vi "Fire_Motor.vi"   [LabVIEW 2011]
uses:
  StateMachineType.ctl
  Robot Global Data.vi
types:
  T1 = typedef "StateMachineType.ctl" = enum16{"Init", "Idle", "Start", "Do", "Stop"}
  T2 = typedef "WPI_MotorControlDeviceRef.ctl" = cluster{"DeviceStatus":errorcluster, "Type":enum16{"PWM", "CAN"}, "PWM":cluster{"Digital Module":T3, "PWM Channel":T4, "DeadBand":T5}, "CAN":cluster{"Device Number":u8, "Control Mode":T6, "Semaphore":T7, "Max Vout":dbl}, "Invert":bool, "TransformRef":T8, "InvTransformRef":T8}
  T3 = typedef "FPGA_TypedefDigitalModule.ctl" = enum16{"Digital Module 1", "Digital Module 2"}
  T4 = typedef "FPGA_DIOPWMChannel.ctl" = enum8{"PWM 1", "PWM 2", "PWM 3", "PWM 4", "PWM 5", "PWM 6", "PWM 7", "PWM 8", "PWM 9", "PWM 10", "Invalid"}
  T5 = typedef "WPI_PWMDeadband.ctl" = cluster{"Name":string, "maxPositivePwm":i32, "minPositivePwm":i32, "centerPwm":i32, "maxNegativePwm":i32, "minNegativePwm":i32, "angularRange":u16}
  T6 = typedef "WPI_CANJaguar_ControlMode.ctl" = enum8{"Percent VBus", "Current", "Speed", "Position", "Voltage"}
  T7 = typedef "Semaphore RefNum" = refnum<k1>
  T8 = typedef "WPI_PWMTransform_ConPane.ctl" = refnum<vi>
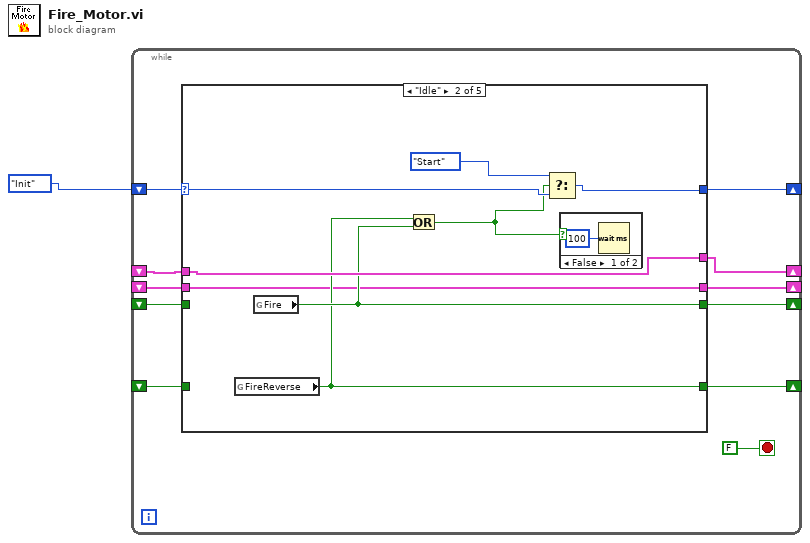
[diagram p0: block diagram]
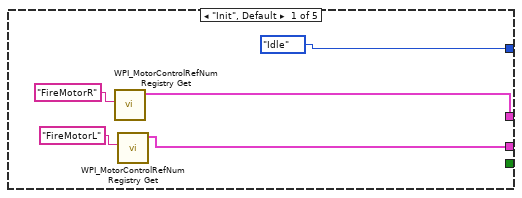
[diagram p2: hidden frame]
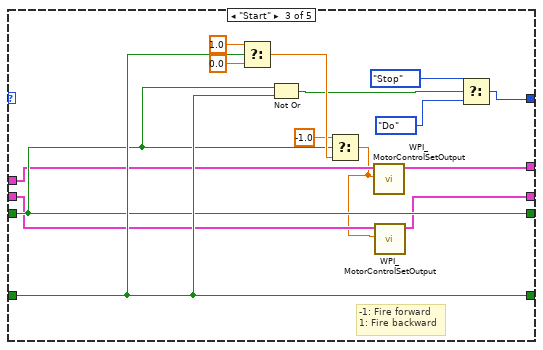
[diagram p4: hidden frame]
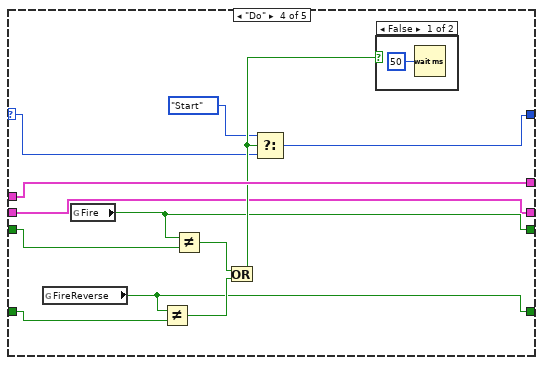
[diagram p5: hidden frame]
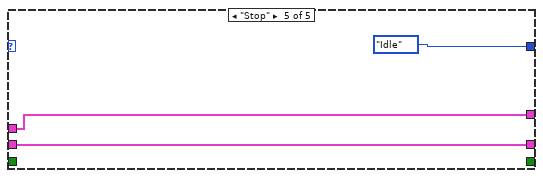
[diagram p7: hidden frame]
diagram:
  n1 = while {
    shift-right: [w8] -> _
    shift-left: _ -> [w11]
    shift-right: [w9] -> _
    shift-left: StateMachineType."Init" -> [w10]
    shift-right: [w6] -> _
    shift-left: _ -> [w4]
    shift-right: [w7] -> _
    shift-left: _ -> [w5]
    shift-right: [w3] -> _
    shift-left: _ -> [w2]
    stop <- FALSE stop-if-true
    n2 = case shown="\"Idle\"" w10 {
      selector: w10 -> [_ w25 _ w43 _]
      tunnel: w11 -> [_ w22 w30 w53 w56]
      tunnel: [StateMachineType."Idle" ("Enum") w23 w37 w47 StateMachineType."Idle" ("Enum")] -> w9
      tunnel: [w15 w22 w41 w53 w56] -> w8
      tunnel: [_ w20 w34 w46 _] -> w7
      tunnel: [_ w19 w35 w45 _] -> w6
      tunnel: w5 -> [_ _ w34 w52 _]
      tunnel: w4 -> [_ _ w35 w51 _]
      tunnel: [w13 w18 w28 w42 w55] -> w3
      tunnel: w2 -> [_ w18 w29 w42 w55]
      frame "Init", Default {
        n3 = call <vilib>:"WPI_MotorControlRefNum Registry Get.vi"("refnum name"="FireMotorR") -> ("MotorControlDevRef"=w15:T2)  [unwired: 9 in, 1 out]
        n4 = call <vilib>:"WPI_MotorControlRefNum Registry Get.vi"("refnum name"="FireMotorL") -> ("MotorControlDevRef"=w13:T2)  [unwired: 9 in, 1 out]
      }
      frame "Idle" {
        n5 = global read "Robot Global Data.vi" "FireReverse"() -> (w19:bool)
        n6 = global read "Robot Global Data.vi" "Fire"() -> (w20:bool)
        n7 = Or(x=w19, y=w20) -> (x .or. y?=w21:bool)
        n8 = Select(t=StateMachineType."Start" ("Enum"), s=w21, f=w25) -> (s? t:f=w23:T1)
        n9 = case shown="False" w21 {
          frame False {
            n10 = Wait (ms)(milliseconds to wait=u32 100) -> ()  [unwired: 1 out]
          }
          frame True {
          }
        }
      }
      frame "Start" {
        # "-1: Fire forward\n1: Fire backward"
        n11 = Select(t=1.0, s=w35, f=0.0) -> (s? t:f=w40:dbl)
        n12 = Not Or(1:w35, 2:w34) -> (0:w36:bool)
        n13 = Select(t=-1.0, s=w34, f=w40) -> (s? t:f=w27:dbl)
        n14 = call <vilib>:"WPI_MotorControlSetOutput.vi"("Output"=w27, "MotorControlDevRef"=w30) -> ("MotorControlDevRef"=w41:T2)  [unwired: 8 in, 1 out]
        n15 = call <vilib>:"WPI_MotorControlSetOutput.vi"("Output"=w27, "MotorControlDevRef"=w29) -> ("MotorControlDevRef"=w28:T2)  [unwired: 8 in, 1 out]
        n16 = Select(t=StateMachineType."Stop" ("Enum"), s=w36, f=StateMachineType."Do" ("Enum")) -> (s? t:f=w37:T1)
      }
      frame "Do" {
        n17 = global read "Robot Global Data.vi" "FireReverse"() -> (w45:bool)
        n18 = global read "Robot Global Data.vi" "Fire"() -> (w46:bool)
        n19 = Not Equal?(x=w45, y=w51) -> (x != y?=w49:bool)
        n20 = Not Equal?(x=w46, y=w52) -> (x != y?=w50:bool)
        n21 = Or(x=w50, y=w49) -> (x .or. y?=w48:bool)
        n22 = Select(t=StateMachineType."Start" ("Enum"), s=w48, f=w43) -> (s? t:f=w47:T1)
        n23 = case shown="False" w48 {
          frame False {
            n24 = Wait (ms)(milliseconds to wait=u32 50) -> ()  [unwired: 1 out]
          }
          frame True {
          }
        }
      }
      frame "Stop" {
      }
    }
  }
